vi "DWF MSO Configure Analog Channel Characteristics.vi"(0 "Instrument Handle In":u32, 5 "Channel":string, 7 "Input Impedance":i32(ring) items=["1 mega ohm", "50 ohms"], 9 "Bandwidth Limit":dbl, 11 "Error In":errorcluster caption="Error In (no error)") -> (4 "Instrument Handle Out":u32, 15 "Error Out":errorcluster)   [LabVIEW 2015, in "DigilentWF.lvlib"]
uses:
  <vilib>/DigilentWF/DigilentWF.lvlib
  dwf.dll
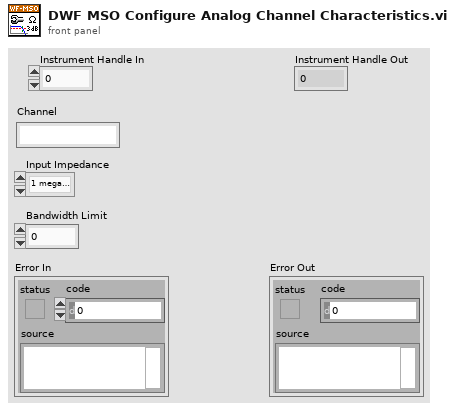
[diagram p1: front panel]
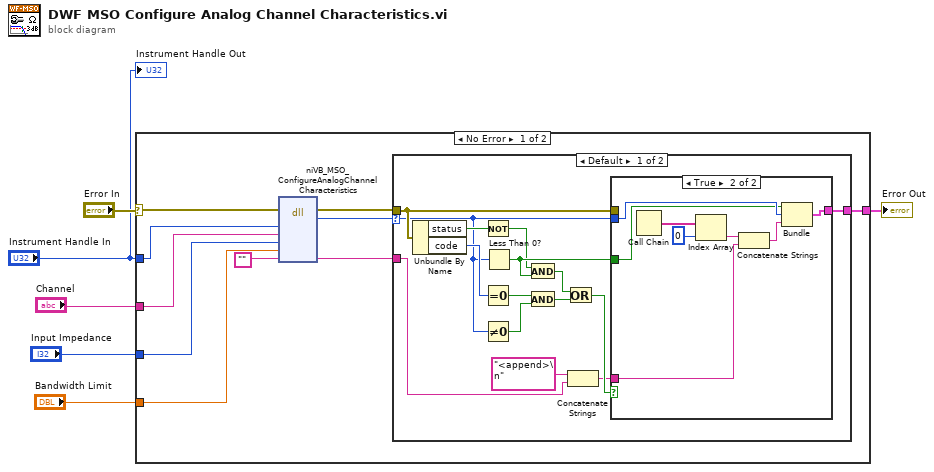
[diagram p0: block diagram]
diagram:
  n1 = case "outter_case" shown="No Error" "Error In" {
    selector: "Error In" -> [w15 w42]
    tunnel: [w16 w42] -> w5
    tunnel: "Instrument Handle In" -> [w13 _]
    tunnel: "Channel" -> [w12 _]
    tunnel: "Input Impedance" -> [w11 _]
    tunnel: "Bandwidth Limit" -> [w10 _]
    frame No Error {
      n2 = dll-call lib="dwf.*" fn="niVB_MSO_ConfigureAnalogChannelCharacteristics"(error in=w15, "instrumentHandle"=w13, "channel"=w12, "inputImpedance"=w11, "bandwidthLimit"=w10, "szError"="") -> (error out=w14:errorcluster, "return type"=w9:u32, "szError"=w7:string)  [unwired: 6 in, 1 out]
      n3 = case "inner_case" shown="Default" w9 {
        selector: w9 -> [w21 _]
        tunnel: w14 -> [w22 w41]
        tunnel: [w18 w41] -> w16
        tunnel: w7 -> [w17 _]
        frame Default {
          n4 = Unbundle By Name(w22) -> ("status"=w26:bool, "code"=w30:i32)
          n5 = Not(x=w26) -> (.not. x?=w29:bool)
          n6 = Equal To 0?(x=w30) -> (x = 0?=w25:bool)
          n7 = Not Equal To 0?(x=w21) -> (x != 0?=w28:bool)
          n8 = Less Than 0?(x=w21) -> (x < 0?=w31:bool)
          n9 = And(x=w29, y=w31) -> (x .and. y?=w27:bool)
          n10 = And(x=w25, y=w28) -> (x .and. y?=w24:bool)
          n11 = Or(x=w27, y=w24) -> (x .or. y?=w23:bool)
          n12 = Concatenate Strings("<append>\n" ("string"), w17) -> (w20:string)
          n13 = case shown="True" w23 {
            tunnel: [w32 w39] -> w18
            tunnel: w21 -> [_ w38]
            tunnel: w31 -> [_ w37]
            tunnel: w22 -> [w32 _]
            tunnel: w20 -> [_ w33]
            frame False {
            }
            frame True {
              n14 = Call Chain() -> (call chain=w36:string[])
              n15 = Index Array(array=w36, index=0) -> (element=w35:string)
              n16 = Concatenate Strings(w35, w33) -> (w40:string)
              n17 = Bundle(w37, "return type"=w38, w40) -> (w39:cluster{bool, "return type":u32, string})  [unwired: 1 out]
            }
          }
        }
        frame 0 {
        }
      }
    }
    frame Error {
    }
  }
  "Error Out" <- w5
  "Instrument Handle Out" <- "Instrument Handle In"
